vi "RSNRPZ Set Auto Max Measuring Time.vi"(8 "error in (no error)":errorcluster, 9 "Upper Time Limit (4.0 s)":dbl=4.0 format="%.2p", 10 "Channel (1)":i32=1, 11 "VISA session":refnum<visa-resource-name> caption="VISA resource name") -> (0 "error out":errorcluster, 3 "dup VISA session":refnum<visa-resource-name> caption="VISA resource name")   [LabVIEW 2010]
doc: "This VI sets an upper time limit can be set via (maximum time). It should never be exceeded. Undesired long measurement times can thus be prevented if the automatic filter length switchover is on.\n\nRemote-control command(s):\nSENS:AVER:COUN:AUTO:MTIM"
uses:
  rsnrpz_32.dll
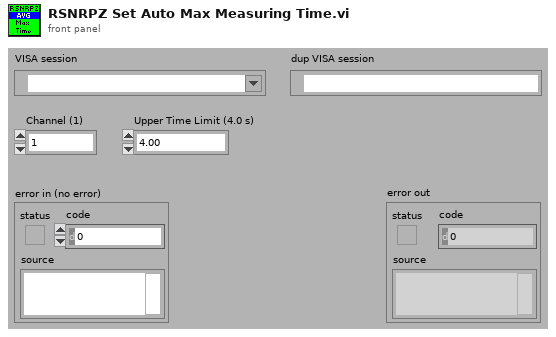
[diagram p1: front panel]
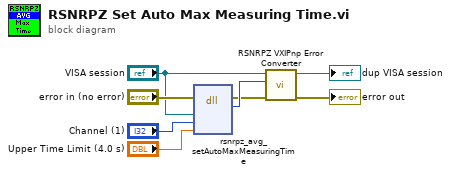
[diagram p0: block diagram]
diagram:
  n1 = dll-call lib="rsnrpz_32.dll" fn="rsnrpz_avg_setAutoMaxMeasuringTime"(error in="error in (no error)", "VISA Session"="VISA session", "Channel"="Channel (1)", "Upper Time Limit"="Upper Time Limit (4.0 s)") -> (error out=w5:errorcluster, "Status"=w8:i32)  [unwired: 5 in, 1 out]
  n2 = call <instrlib>:"RSNRPZ VXIPnp Error Converter.vi"("error in"=w5, "VXIPnp error code"=w8, "VISA session"="VISA session") -> ("error out"=→"error out":errorcluster, "dup VISA session"=→"dup VISA session":refnum<visa-resource-name>)  [unwired: 7 in]
